vi "Clear IP.vi"(8 "error in (no error)":errorcluster, 11 "Digital Pattern Generation in":refnum<class "Digital Pattern Generation.lvclass">) -> (0 "error out":errorcluster)   [LabVIEW 2013, in "Digital Pattern Generation.lvclass"]
uses:
  Digital Pattern Generation.lvclass
  Engine Simulation IP.lvclass
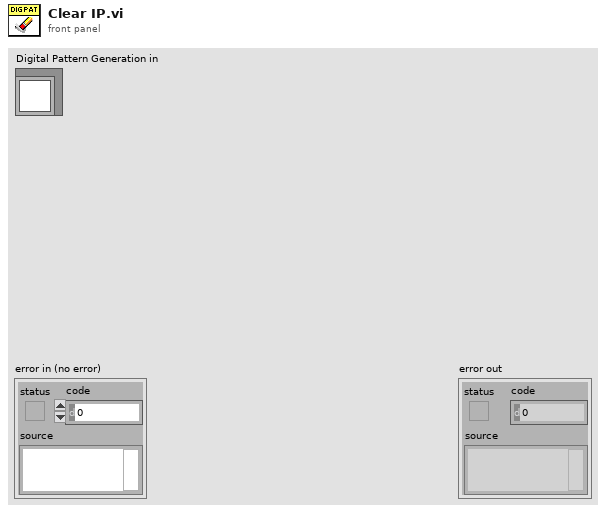
[diagram p1: front panel]
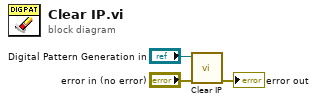
[diagram p0: block diagram]
diagram:
  n1 = call-parent "Clear IP.vi"("error in (no error)"="error in (no error)", "Engine Simulation IP in"="Digital Pattern Generation in") -> ("error out"=→"error out":errorcluster)  [unwired: 9 in]
